vi "power-fit.vi"() -> ()   [LabVIEW 2014]
panel:
  in  "Powers":dbl[](graph)=[0.00279, 0.002982, 0.002782, 0.002538, 0.001682, 0.00174, 0.002118, 0.001765, 0.00142, 0.001148, 0.000401, 0.000503, 0.000803, 0.00122, 0.001047, 0.001043, 0.00127, 0.001892, 0.002092, 0.002645, 0.002642, 0.002781, 0.002918, 0.003173, 0.003136, 0.003731, 0.00354, 0.003536, 0.003714, 0.003515, 0.003254, 0.002968, 0.003428, 0.005023, 0.005137, 0.005979, 0.005696, 0.005479, 0.005892, 0.006487, 0.005314, 0.005488, 0.006165, 0.006447, 0.006529, 0.006884, 0.006302, 0.006191, 0.006613, 0.006996, 0.006434, 0.005925, 0.006298, 0.006737, 0.006851, 0.007169, 0.00749, 0.007571, 0.007879, 0.007998, 0.008451, 0.00878, 0.008868, 0.009089, 0.008981, 0.008982, 0.009346, 0.009209, 0.010035, 0.009883, 0.010295, 0.010508, 0.010774, 0.010903, 0.010857, 0.010079, 0.010241, 0.010333, 0.010278, 0.009975, 0.009731, 0.009657, 0.01064, 0.010531, 0.008393, 0.00806, 0.00871, 0.008561, 0.009385, 0.010971, 0.010026, 0.010356, 0.01061, 0.010615, 0.010928, 0.010942, 0.01071, 0.01064, 0.010612, 0.011328, 0.012453, 0.01262, 0.012773, 0.013068, 0.013342]
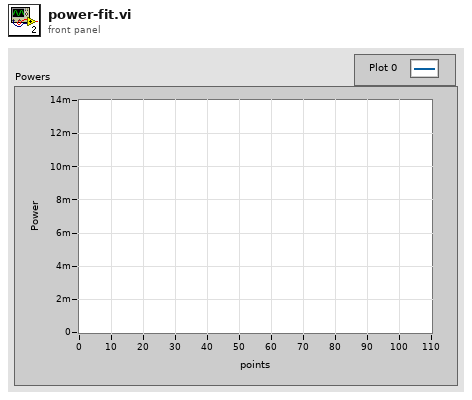
[diagram p1: front panel]
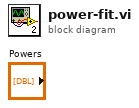
[diagram p0: block diagram]
diagram:
